vi "Configure Modulation Duty Cycle.vi"(8 "error in (no error)":errorcluster, 10 "duty cycle, %":dbl=50.0, 11 "HFP Gen in":refnum<class "PL HFP Generator.lvclass">) -> (0 "error out":errorcluster, 3 "HFP Gen out":refnum<class "PL HFP Generator.lvclass">)   [LabVIEW 2015, in "PL HFP Generator.lvclass"]
doc: "Configures modulation duty cycle."
uses:
  PL HFP Generator.lvclass
  PL HFP Generator.lvclass/PL HFP Generator.ctl
  <vilib>/plasmapper/PL Modbus Client/PL Modbus Client.lvclass
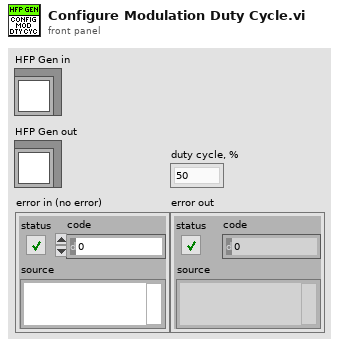
[diagram p1: front panel]
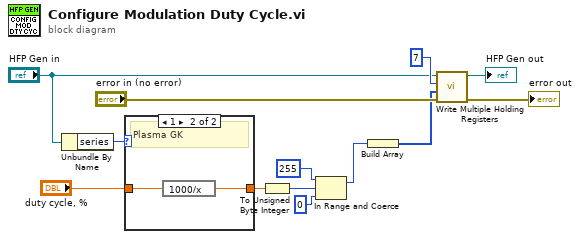
[diagram p0: block diagram]
diagram:
  n1 = Unbundle By Name("HFP Gen in") -> ("series"=w7:u16)
  n2 = case shown="1" w7 {
    tunnel: "duty cycle, %" -> [w14 w16]
    tunnel: [w14 w15] -> w6
    frame 0, Default {
      # "Plasma G20"
    }
    frame 1 {
      # "Plasma GK"
      n3 = expression code="1000/x"(w16) -> (w15:dbl)
    }
  }
  n4 = To Unsigned Byte Integer(number=w6) -> (unsigned 8bit integer=w5:u8)
  n5 = In Range and Coerce(upper limit=u8 255, x=w5, lower limit=u8 0) -> (coerced(x)=w4:u8)  [unwired: 1 out]
  n6 = Build Array(w4) -> (w2:u8[])
  n7 = call <vilib>:"Write Multiple Holding Registers.vi"("error in (no error)"="error in (no error)", "values"=w2, "address"=u16 7, "MODBUS in"="HFP Gen in") -> ("error out"=→"error out":errorcluster, "MODBUS out"=→"HFP Gen out":refnum<class "PL HFP Generator.lvclass">)  [unwired: 6 in]
